vi "Append List to Report.vi"(0 "report in":refnum<class "ooCalc.lvclass">, 1 "ordered item type (default)":T1(ring), 2 "unordered item type (default)":enum16{"(default)", "disc", "square", "circle"}(ring), 7 "list elements":string[](array[string]), 9 "list type (ordered)":enum16{"unordered", "ordered"}(ring)=enum."ordered", 11 "error in (no error)":errorcluster, 12 "ordered start (1)":i32=1, 13 "bookmark (Word)":string) -> (4 "report out":refnum<class "ooCalc.lvclass">, 8 "start out (Word)":i32, 10 "end out (Word)":i32, 15 "error out":errorcluster)   [LabVIEW 2009, in "ooCalc.lvclass"]
doc: "Adds a list of elements to the report."
uses:
  ooCalc.lvclass
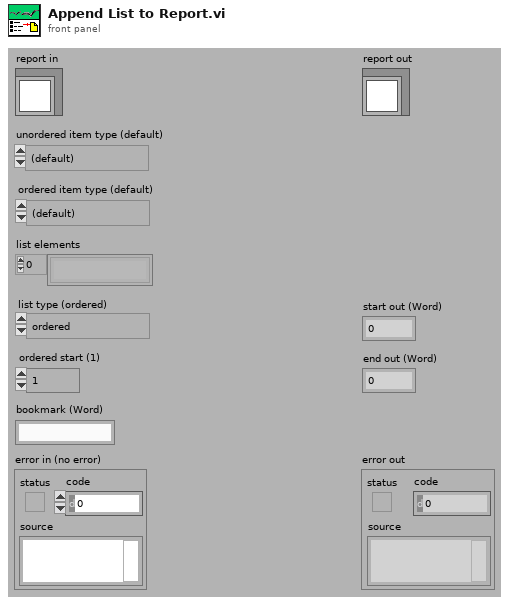
[diagram p1: front panel]
types:
  T1 = enum16{"(default)", "arabic numerals", "lower alpha", "upper alpha"}
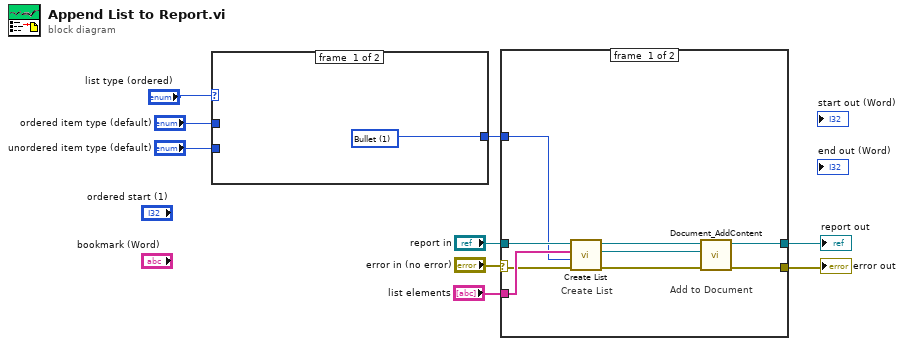
[diagram p0: block diagram]
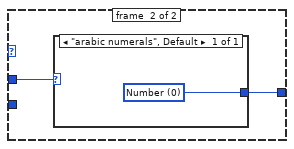
[diagram p2: hidden frame]
diagram:
  n1 = case shown="\"ordered\"" "list type (ordered)" {
    tunnel: "ordered item type (default)" -> [_ w12]
    tunnel: "unordered item type (default)" -> [_ _]
    tunnel: [w10 w11] -> w1
    frame #0 {
      w10 = 1 items=["Number", "Bullet"] ("typ")
    }
    frame #1 {
      n2 = case shown="\"arabic numerals\", Default" w12 {
        tunnel: [w13] -> w11
        frame "arabic numerals", Default {
          w13 = 0 items=["Number", "Bullet"] ("typ")
        }
      }
    }
  }
  n3 = case shown="No Error" "error in (no error)" {
    selector: "error in (no error)" -> [w17 w23]
    tunnel: [w21 w23] -> w8
    tunnel: "report in" -> [w20 w24]
    tunnel: [w22 w24] -> w6
    tunnel: "list elements" -> [w19 _]
    tunnel: w1 -> [w18 _]
    frame #0 {
      # "Create List"
      # "Add to Document"
      n4 = call-dynamic "Create List.vi"("error in (no error)"=w17, "List type"=w18, "list elements"=w19, "ooCalc in"=w20) -> ("error out"=w14:errorcluster, "List"=w15:refnum<k24>, "ooCalc out"=w16:refnum<class "ooCalc.lvclass">)  [unwired: 5 in]
      n5 = call-dynamic "Document_AddContent.vi"("error in (no error)"=w14, "Content"=w15, "ooCalc in"=w16) -> ("error out"=w21:errorcluster, "ooCalc out"=w22:refnum<class "ooCalc.lvclass">)  [unwired: 7 in]
    }
    frame #1 {
    }
  }
  "error out" <- w8
  "report out" <- w6
